vi "Set Parent Name.vi"(8 "error in (no error)":errorcluster, 10 "Parent Name":string, 11 "DataHandlerTask in":refnum<class "DataHandlerTask.lvclass">) -> (0 "error out":errorcluster, 3 "DataHandlerTask out":refnum<class "DataHandlerTask.lvclass">)   [LabVIEW 2020, in "Volatus.lvlib" / "DataHandlerTask.lvclass"]
uses:
  DataHandlerTask.lvclass
  DataHandlerTask.lvclass/DataHandlerTask.ctl
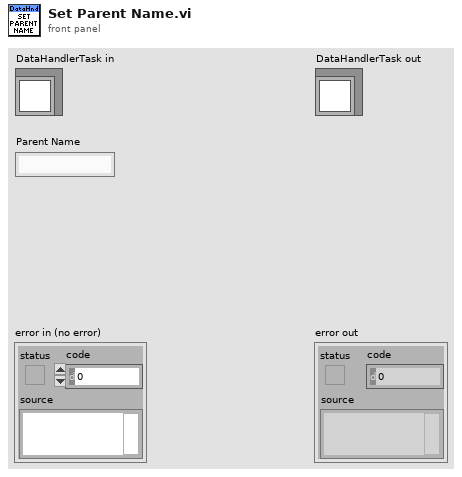
[diagram p1: front panel]
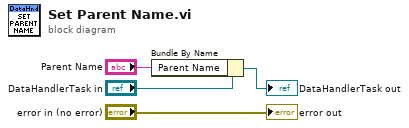
[diagram p0: block diagram]
diagram:
  n1 = Bundle By Name(cluster="DataHandlerTask in", "Parent Name"="Parent Name") -> (→"DataHandlerTask out":refnum<class "DataHandlerTask.lvclass">)
  "error out" <- "error in (no error)"
